vi "Untitled 10.vi"() -> ()   [LabVIEW 2019]
uses:
  Generated_client/RPC Messages/Greeter_req.ctl
  Generated_client/RPC Messages/Greeter_req_req_oneof/Greeter_req_req_oneof.lvclass
  Generated_client/RPC Messages/Greeter_Color.ctl
  Generated_client/RPC Messages/Greeter_req_req_oneof/Greeter_req_req_oneof.lvclass/Greeter_req_req_oneof.ctl
  Generated_client/RPC Messages/Greeter_res_res_oneof/Greeter_res_res_oneof.lvclass/Greeter_res_res_oneof.ctl
  Generated_client/Generated_client.lvlib
  Generated_client/RPC Messages/Greeter_res_res_oneof/Greeter_res_res_oneof.lvclass
panel:
  out "Has Data?":bool
  out "Get_Val":T1
  in  "Set_Val":T1
  out "res_latitude":i32
  out "error out":errorcluster
  in  "Request Data":T2
  in  "address":string
  in  "error in":errorcluster
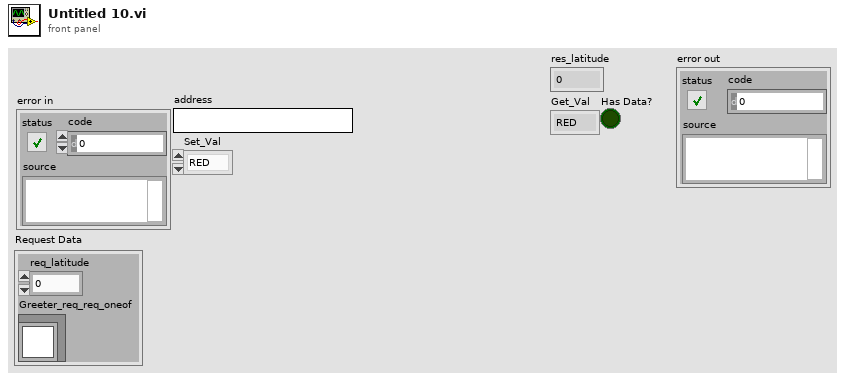
[diagram p1: front panel]
types:
  T1 = typedef "Generated_client.lvlib/Greeter_Color.ctl" = enum32{"RED", "GREEN", "BLUE"}
  T2 = typedef "Generated_client.lvlib/Greeter_req.ctl" = cluster{"req_latitude":i32, "Greeter_req_req_oneof":refnum<class "Greeter_req_req_oneof.lvclass">}
  T3 = typedef "grpc-lvsupport-release.lvlib/grpcId.ctl" = u64
  T4 = typedef "Generated_client.lvlib/Greeter_res.ctl" = cluster{"res_latitude":i32, "Greeter_res_res_oneof":refnum<class "Greeter_res_res_oneof.lvclass">}
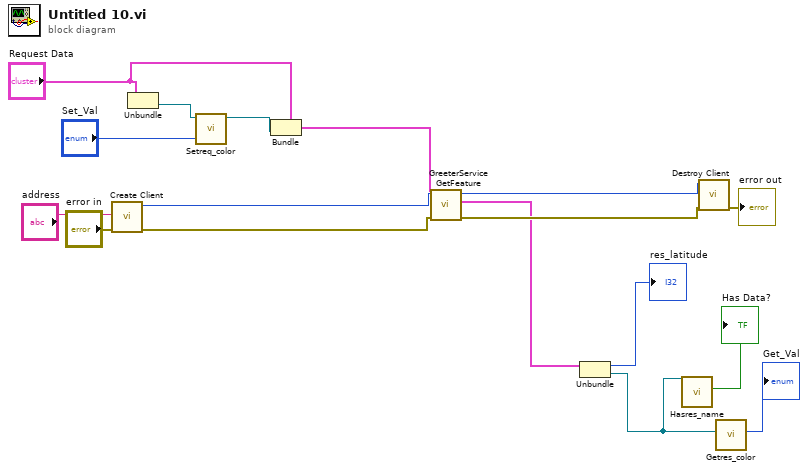
[diagram p0: block diagram]
diagram:
  n1 = call "Create Client.vi"("error in"="error in", "address"="address") -> ("error out"=w15:errorcluster, "gRPC ID Out"=w17:T3)  [unwired: 8 in]
  n2 = Unbundle("Request Data") -> ("Greeter_req_req_oneof"=w6:refnum<class "Greeter_req_req_oneof.lvclass">)  [unwired: 1 out]
  n3 = call "Setreq_color.vi"("Set_Val"="Set_Val", "OneOfTemplate in"=w6) -> ("OneOfTemplate out"=w4:refnum<class "Greeter_req_req_oneof.lvclass">)  [unwired: 8 in, 1 out]
  n4 = Bundle(cluster="Request Data", "Greeter_req_req_oneof"=w4) -> (w9:T2)  [unwired: 1 in]
  n5 = call "GreeterService GetFeature.vi"("error in"=w15, "Request Data"=w9, "gRPC ID"=w17) -> ("error out"=w14:errorcluster, "Response Data"=w8:T4, "gRPC ID out"=w16:T3)  [unwired: 6 in]
  n6 = Unbundle(w8) -> ("res_latitude"=→"res_latitude":i32, "Greeter_res_res_oneof"=w2:refnum<class "Greeter_res_res_oneof.lvclass">)
  n7 = call "Hasres_name.vi"("OneOfTemplate in"=w2) -> ("Has Data?"=→"Has Data?":bool)  [unwired: 8 in, 2 out]
  n8 = call "Destroy Client.vi"("error in"=w14, "gRPC ID"=w16) -> ("error out"=→"error out":errorcluster)  [unwired: 9 in]
  n9 = call "Getres_color.vi"("OneOfTemplate in"=w2) -> ("Get_Val"=→"Get_Val":T1)  [unwired: 8 in, 2 out]
